vi "MicrometerGlue.vi"() -> ()   [LabVIEW 2015]
uses:
  <vilib>/Analysis/5stat.llb/RMS (DBL).vi
  <vilib>/Analysis/baseanly.llb/Mean (DBL).vi
  <vilib>/Utility/file.llb/Read From Spreadsheet File (DBL).vi
  <vilib>/Analysis/NI_AALPro.lvlib
  <vilib>/Analysis/NI_AALBase.lvlib
panel:
  out "x         y       DR      Meas   Diff":dbl[][](array[numeric]) format="%#_4f"
  out "nome file":string="micrometer_"
  in  "suffisso (se necessario)":string
  out "rms value":dbl format="%0.2f"
  out "mean":dbl format="%0.2f"
  out "appended array":dbl[](array[numeric])
  in  "stop":bool
  in  "2200,500":dbl format="%.2g"
  in  "2200,400":dbl format="%.2g"
  in  "0,500":dbl format="%.2g"
  in  "0,400":dbl format="%.2g"
  in  "2000,200":dbl format="%.2g"
  in  "1550,200":dbl format="%.2g"
  in  "1200,200":dbl format="%.2g"
  in  "800,200":dbl format="%.2g"
  in  "200,200":dbl format="%.2g"
  in  "2000,1100":dbl format="%.2g"
  in  "1550,1100":dbl format="%.2g"
  in  "1200, 1100":dbl format="%.2g"
  in  "800,1100":dbl format="%.2g"
  in  "200,1100":dbl format="%.2g"
  # "Dopo Incollaggio"
  # "- Scrivi i valori delle misure effettuate con il micrometro nelle                                  caselle corrispondenti\n- Aggiungi il suffisso al nome del file (se necessario)\n- clicca su \"DONE\" quando hai immesso tutti i valori"
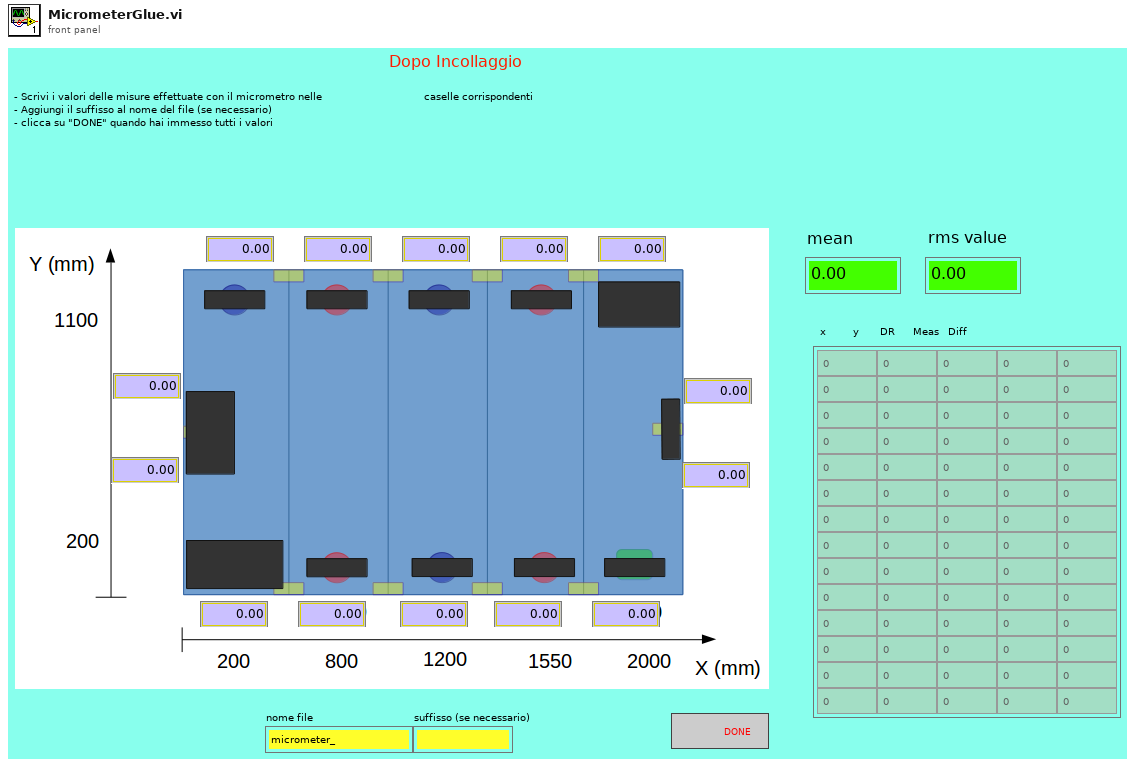
[diagram p1: front panel]
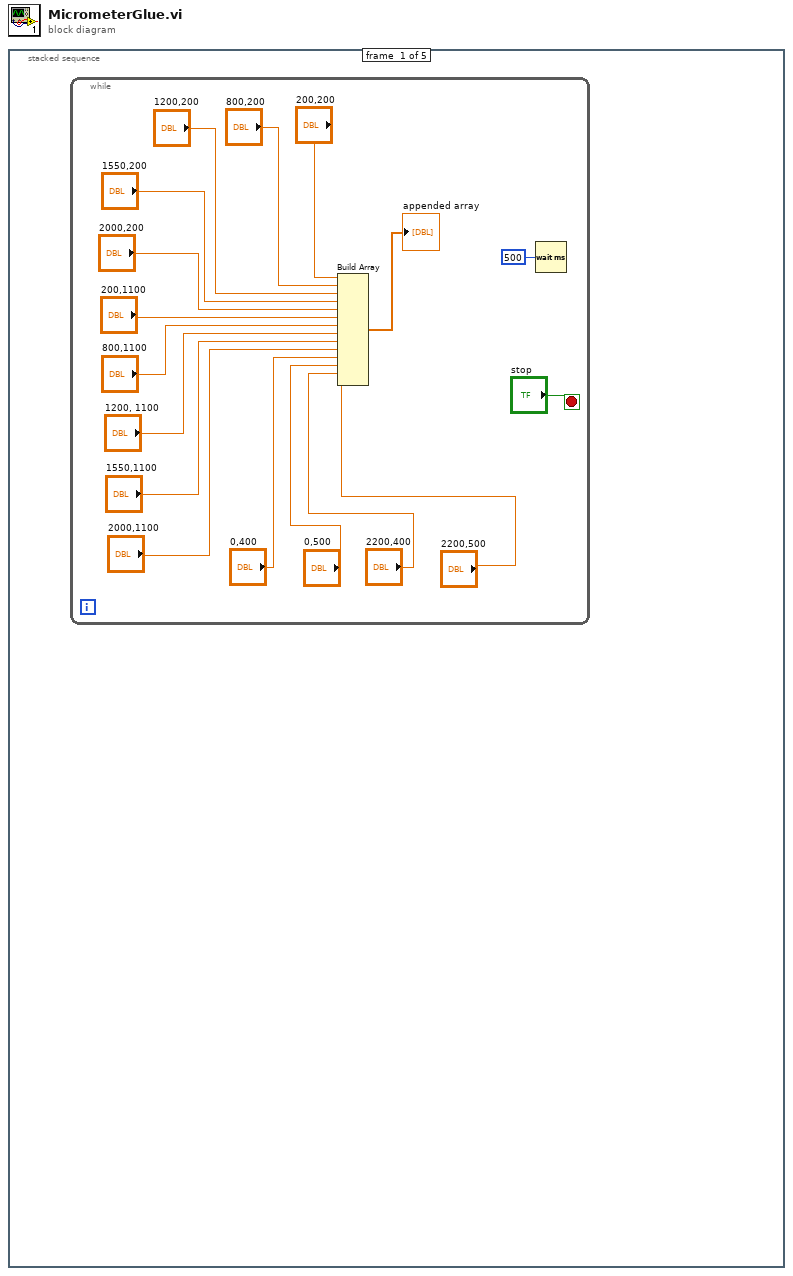
[diagram p0: block diagram]
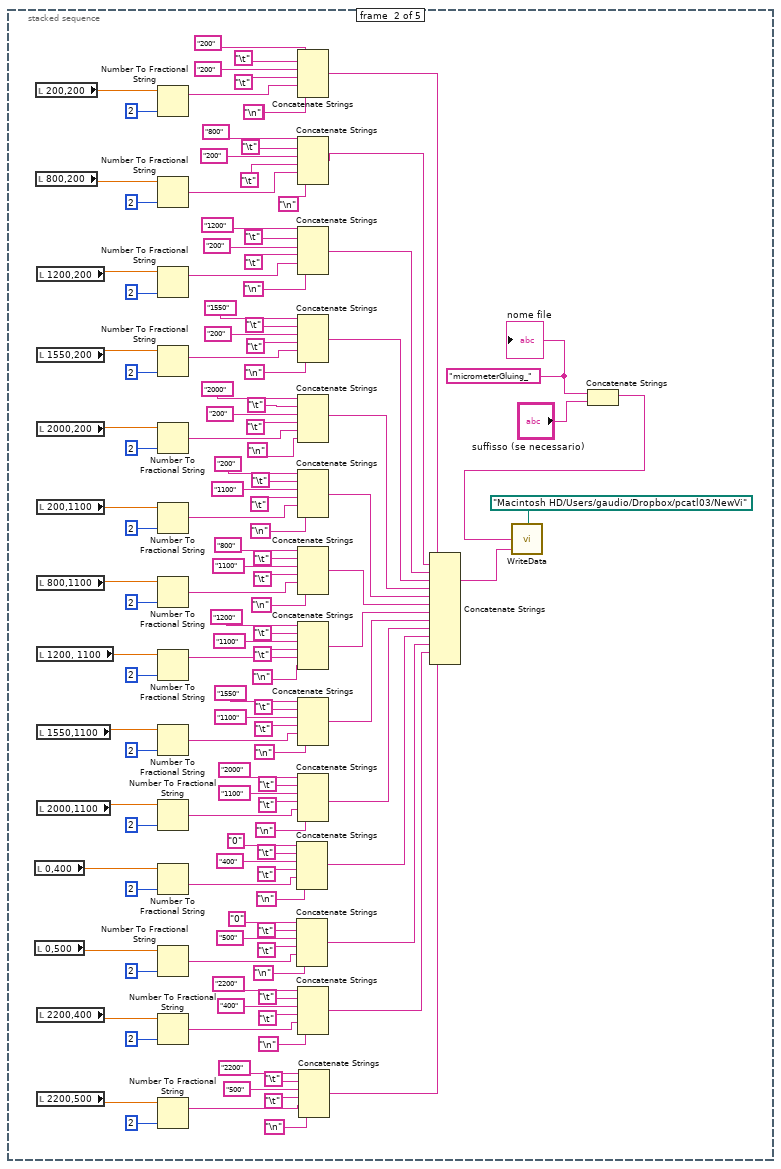
[diagram p2: hidden frame]
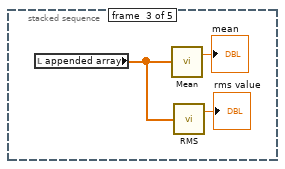
[diagram p3: hidden frame]
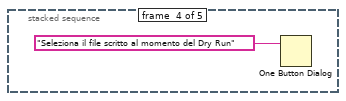
[diagram p4: hidden frame]
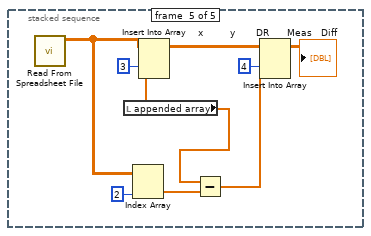
[diagram p5: hidden frame]
diagram:
  n1 = stacked-sequence {
    frame #0 {
      n2 = while {
        stop <- "stop" stop-if-true
        n3 = Build Array("200,200", "800,200", "1200,200", "1550,200", "2000,200", "200,1100", "800,1100", "1200, 1100", "1550,1100", "2000,1100", "0,400", "0,500", "2200,400", "2200,500") -> (→"appended array":dbl[])
        n4 = Wait (ms)(milliseconds to wait=u32 500) -> ()  [unwired: 1 out]
      }
    }
    frame #1 {
      w20 = "micrometerGluing_" ("string")
      (unwired) "\n"
      n5 = local read "0,400"() -> (w45:dbl)
      n6 = local read "0,500"() -> (w44:dbl)
      n7 = local read "200,200"() -> (w134:dbl)
      n8 = local read "800,200"() -> (w133:dbl)
      n9 = local read "1200,200"() -> (w111:dbl)
      n10 = local read "1550,200"() -> (w110:dbl)
      n11 = local read "2000,200"() -> (w109:dbl)
      n12 = local read "200,1100"() -> (w74:dbl)
      n13 = local read "800,1100"() -> (w73:dbl)
      n14 = local read "1200, 1100"() -> (w72:dbl)
      n15 = local read "1550,1100"() -> (w71:dbl)
      n16 = local read "2000,1100"() -> (w70:dbl)
      n17 = local read "2200,400"() -> (w43:dbl)
      n18 = local read "2200,500"() -> (w42:dbl)
      n19 = Number To Fractional String(number=w134, precision (6)=i16 2) -> (F-format string=w143:string)  [unwired: 2 in]
      n20 = Number To Fractional String(number=w133, precision (6)=i16 2) -> (F-format string=w137:string)  [unwired: 2 in]
      n21 = Number To Fractional String(number=w111, precision (6)=i16 2) -> (F-format string=w120:string)  [unwired: 2 in]
      n22 = Number To Fractional String(number=w110, precision (6)=i16 2) -> (F-format string=w126:string)  [unwired: 2 in]
      n23 = Number To Fractional String(number=w109, precision (6)=i16 2) -> (F-format string=w132:string)  [unwired: 2 in]
      n24 = Number To Fractional String(number=w74, precision (6)=i16 2) -> (F-format string=w108:string)  [unwired: 2 in]
      n25 = Number To Fractional String(number=w73, precision (6)=i16 2) -> (F-format string=w101:string)  [unwired: 2 in]
      n26 = Number To Fractional String(number=w72, precision (6)=i16 2) -> (F-format string=w83:string)  [unwired: 2 in]
      n27 = Number To Fractional String(number=w71, precision (6)=i16 2) -> (F-format string=w90:string)  [unwired: 2 in]
      n28 = Number To Fractional String(number=w70, precision (6)=i16 2) -> (F-format string=w80:string)  [unwired: 2 in]
      n29 = Number To Fractional String(number=w45, precision (6)=i16 2) -> (F-format string=w69:string)  [unwired: 2 in]
      n30 = Number To Fractional String(number=w44, precision (6)=i16 2) -> (F-format string=w63:string)  [unwired: 2 in]
      n31 = Number To Fractional String(number=w43, precision (6)=i16 2) -> (F-format string=w51:string)  [unwired: 2 in]
      n32 = Number To Fractional String(number=w42, precision (6)=i16 2) -> (F-format string=w57:string)  [unwired: 2 in]
      n33 = Concatenate Strings("0", "\t", "400", "\t", w69, "\n") -> (w26:string)
      n34 = Concatenate Strings("0", "\t", "500", "\t", w63, "\n") -> (w25:string)
      n35 = Concatenate Strings("200", "\t", "200", "\t", w143, "\n") -> (w36:string)
      n36 = Concatenate Strings("800", "\t", "200", "\t", w137, "\n") -> (w35:string)
      n37 = Concatenate Strings("1200", "\t", "200", "\t", w120, "\n") -> (w34:string)
      n38 = Concatenate Strings("1550", "\t", "200", "\t", w126, "\n") -> (w33:string)
      n39 = Concatenate Strings("2000", "\t", "200", "\t", w132, "\n") -> (w32:string)
      n40 = Concatenate Strings("200", "\t", "1100", "\t", w108, "\n") -> (w31:string)
      n41 = Concatenate Strings("800", "\t", "1100", "\t", w101, "\n") -> (w30:string)
      n42 = Concatenate Strings("1200", "\t", "1100", "\t", w83, "\n") -> (w29:string)
      n43 = Concatenate Strings("1550", "\t", "1100", "\t", w90, "\n") -> (w28:string)
      n44 = Concatenate Strings("2000", "\t", "1100", "\t", w80, "\n") -> (w27:string)
      n45 = Concatenate Strings("2200", "\t", "400", "\t", w51, "\n") -> (w24:string)
      n46 = Concatenate Strings("2200", "\t", "500", "\t", w57, "\n") -> (w23:string)
      n47 = Concatenate Strings(w36, w35, w34, w33, w32, w31, w30, w29, w28, w27, w26, w25, w24, w23) -> (w18:string)
      n48 = Concatenate Strings(w20, "suffisso (se necessario)") -> (w21:string)
      n49 = call "WriteData.vi"("Message"=w18, "File Prefix"=w21, "base path"=path "/Macintosh HD/Users/gaudio/Dropbox/pcatl03/NewVi") -> ()
      "nome file" <- w20
    }
    frame #2 {
      n50 = local read "appended array"() -> (w149:dbl[])
      n51 = call-poly <vilib>:"Mean.vi"("X"=w149) -> ("mean"=→"mean":dbl)  [unwired: 1 out]
      n52 = call-poly <vilib>:"RMS.vi"("X"=w149) -> ("rms value"=→"rms value":dbl)  [unwired: 1 out]
    }
    frame #3 {
      n53 = One Button Dialog(message="Seleziona il file scritto al momento del Dry Run") -> ()  [unwired: 1 in, 1 out]
    }
    frame #4 {
      n54 = call-poly <vilib>:"Read From Spreadsheet File.vi"() -> ("all rows"=w160:dbl[][])  [unwired: 7 in, 4 out]
      n55 = local read "appended array"() -> (w154:dbl[])
      n56 = Index Array(array=w160, index (col)=2 ("disabled index (col)")) -> (element=w153:dbl[])  [unwired: 1 in]
      n57 = Insert Into Array(array=w160, index (col)=3 ("disabled index (col)"), new element=w154) -> (w158:dbl[][])  [unwired: 1 in]
      n58 = Subtract(x=w154, y=w153) -> (x-y=w157:dbl[])
      n59 = Insert Into Array(array=w158, index (col)=4 ("disabled index (col)"), new element=w157) -> (→"x         y       DR      Meas   Diff":dbl[][])  [unwired: 1 in]
    }
  }
